vi "WriteTxtDataFile_DP_ver1.0.vi"(2 "2D Data Array In":dbl[][](array[numeric]), 3 "Title Name Array":string[](array[string]), 4 "error in":errorcluster, 5 "Run Info. Comment":string, 6 "Initial String":string, 7 "file path":path) -> (0 "error out":errorcluster)   [LabVIEW 2012]
doc: "Input 2D data array and Data Save Info. Then, save all the data and info. in Igor format. If \"Title Name Array\" is empty, the title name in igor file would be the title name column from \"Instrs configs 2D arrary\""
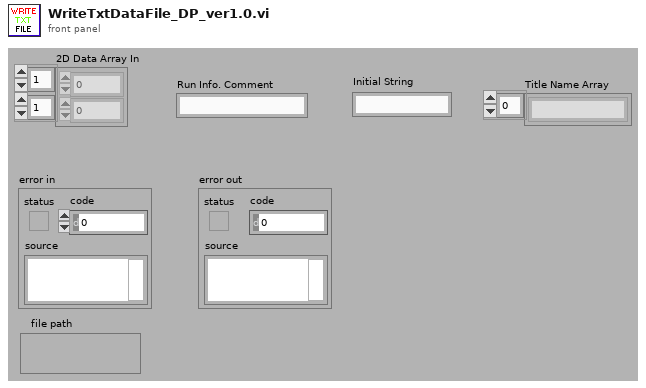
[diagram p1: front panel]
types:
  T1 = enum16{"open", "replace", "create", "open or create", "replace or create", "replace or create with confirmation"}
  T2 = enum16{"open", "open or create", "create or replace", "create", "open (read only)"}
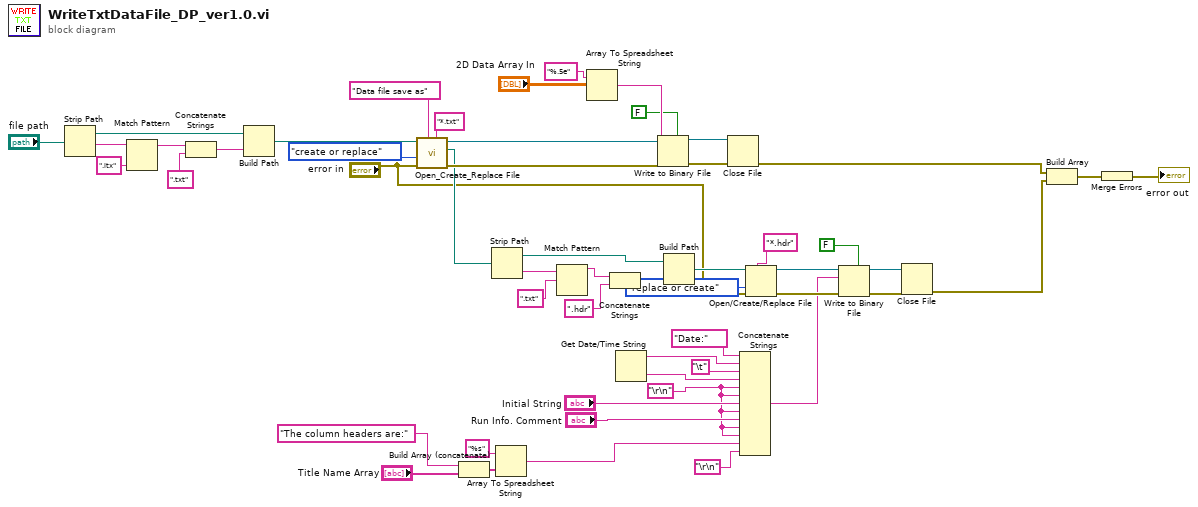
[diagram p0: block diagram]
diagram:
  w1 = "\r\n"
  n1 = Strip Path(path="file path") -> (stripped path=w37:path, name=w44:string)
  n2 = Match Pattern(string=w44, regular expression=".itx") -> (before substring=w38:string)  [unwired: 1 in, 3 out]
  n3 = Concatenate Strings(w38, ".txt" ("format string")) -> (w42:string)
  n4 = Build Path(base path=w37, name or relative path=w42) -> (appended path=w41:path)
  n5 = call <vilib>:"Open_Create_Replace File.vi"("pattern"="*.txt", "prompt"="Data file save as", "error in (no error)"="error in", "function (open:0)"=T2."create or replace", "file path"=w41) -> ("error out"=w39:errorcluster, "new file path"=w36:path, "refnum"=w40:refnum<file>)  [unwired: 2 in, 2 out]
  n6 = Build Array (concatenate)("The column headers are:" ("string"), "Title Name Array") -> (w7:string[])
  n7 = Strip Path(path=w36) -> (stripped path=w30:path, name=w35:string)
  n8 = Array To Spreadsheet String(array=w7, 3:"%s" ("format string")) -> (spreadsheet string=w2:string)  [unwired: 1 out]
  n9 = Match Pattern(string=w35, regular expression=".txt") -> (before substring=w33:string)  [unwired: 1 in, 3 out]
  n10 = Array To Spreadsheet String(array="2D Data Array In", 3:"%.5e" ("format string")) -> (spreadsheet string=w52:string)  [unwired: 1 out]
  n11 = Concatenate Strings(w33, ".hdr" ("format string")) -> (w31:string)
  n12 = Get Date/Time String() -> (date string=w25:string, time string=w23:string)  [unwired: 3 out]
  n13 = Write to Binary File(file (use dialog)=w40, data=w52, error in=w39, 5:FALSE ("prepend array or string size? (T)")) -> (refnum out=w16:refnum<file>, error out=w17:errorcluster)  [unwired: 3 out]
  n14 = Build Path(base path=w30, name or relative path=w31) -> (appended path=w29:path)
  n15 = Close File(refnum=w16, error in=w17) -> (error out=w14:errorcluster)  [unwired: 1 out]
  n16 = Concatenate Strings("Date:" ("string"), w25, "\t", w23, w1, w1, "Initial String", w1, "Run Info. Comment", w1, w1, w2, "\r\n") -> (w19:string)
  n17 = Open/Create/Replace File(file path (use dialog)=w29, error in="error in", prompt="*.hdr" ("pattern"), operation (0:open)=T1."replace or create") -> (refnum out=w21:refnum<file>, error out=w20:errorcluster)  [unwired: 2 in, 1 out]
  n18 = Write to Binary File(file (use dialog)=w21, data=w19, error in=w20, 5:FALSE ("prepend array or string size? (T)")) -> (refnum out=w13:refnum<file>, error out=w12:errorcluster)  [unwired: 3 out]
  n19 = Close File(refnum=w13, error in=w12) -> (error out=w11:errorcluster)  [unwired: 1 out]
  n20 = Build Array(w14, w11) -> (w15:errorcluster[])
  n21 = Merge Errors(w15) -> (→"error out":errorcluster)
